vi "Gif.Main.vi"(5 "String":string, 9 "bgcolor":u32(colorbox)=16777226, 11 "error in (no error)":errorcluster, 12 "image index":i32) -> (6 "time":u32[](array[numeric]), 8 "images out":picture[](array[picture]), 13 "image data":T1, 14 "image size":cluster{"Width":u32, "Height":u32}, 15 "error out":errorcluster)   [LabVIEW 2011]
doc: "This VI reads all images from a gif file.\nCurrently it can only read from version 89a.\nInterlaced images are not taken into account.\n\nThe outputs are an array of all delay times, an array of all images, the image size and an error cluster.\n\nVersion 01.01\nMike Schröder"
uses:
  <vilib>/picture/picture.llb/imagedata.ctl
panel:
  out "color table":u32[](array[colorbox])
  out "Version":string
  out "Signature":string
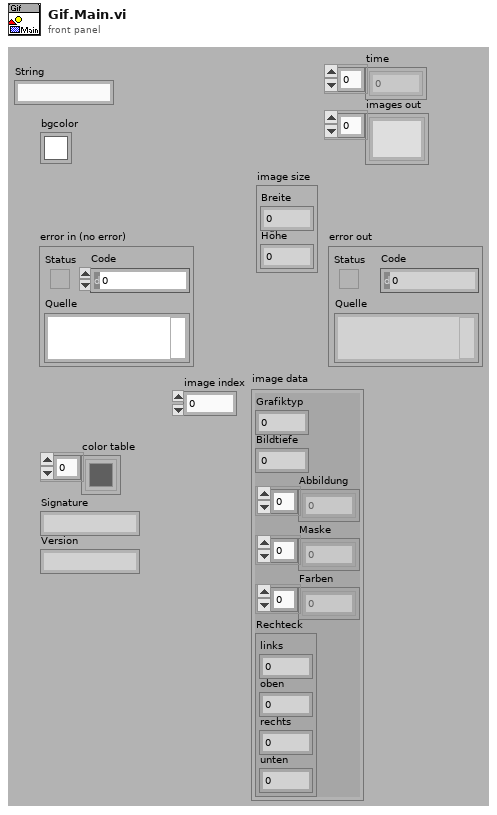
[diagram p1: front panel]
types:
  T1 = typedef "imagedata.ctl" = cluster{"image type":i32, "image depth":i32, "image":u8[], "mask":u8[], "colors":u32[], "Rectangle":cluster{"left":i16, "top":i16, "right":i16, "bottom":i16}}
  T2 = typedef "Gif.LogicalScreenDescriptior.ctl" = cluster{"Logical Screen Width":u16, "Logical Screen Height":u16, "Global Color Table Flag":u8, "Color Resolution":u8, "Sort Flag":u8, "Size of Global Color Table":u8, "Background Color Index":u8, "Pixel Aspect Ratio":u8}
  T3 = typedef "Gif.GraphicControlExtension.ctl" = cluster{"Reserved":u8, "Disposal Method":u8, "User Input Flag":u8, "Transparent Color Flag":u8, "Delay Time":u16, "Transparent Color Index":u8}
  T4 = typedef "Gif.ImageDescriptor.ctl" = cluster{"Image Left Position":u16, "Image Top Position":u16, "Image Width":u16, "Image Height":u16, "Local Color Table Flag":u8, "Interlace Flag":u8, "Sort Flag":u8, "Reserved":u8, "Size Of Local Color Table":u8}
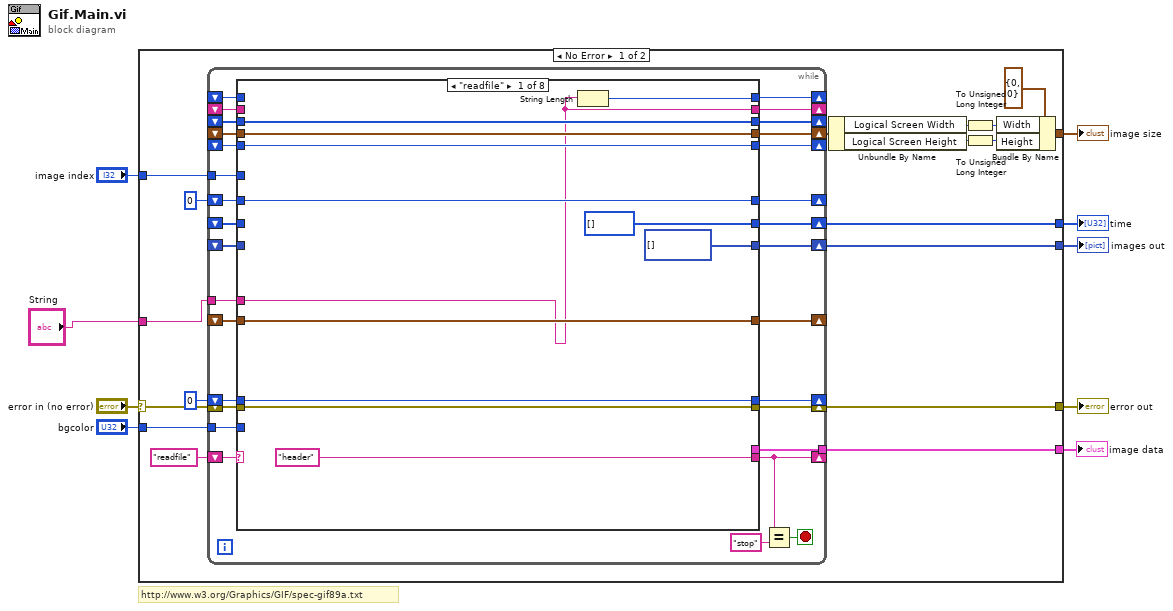
[diagram p0: block diagram]
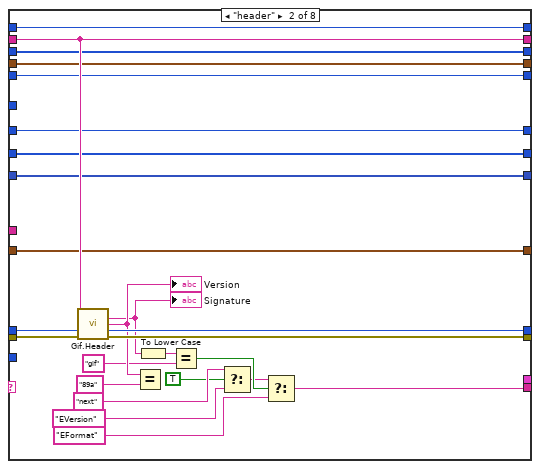
[diagram p2: hidden frame]
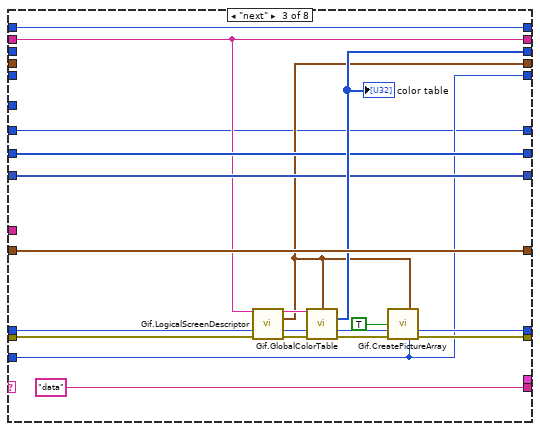
[diagram p3: hidden frame]
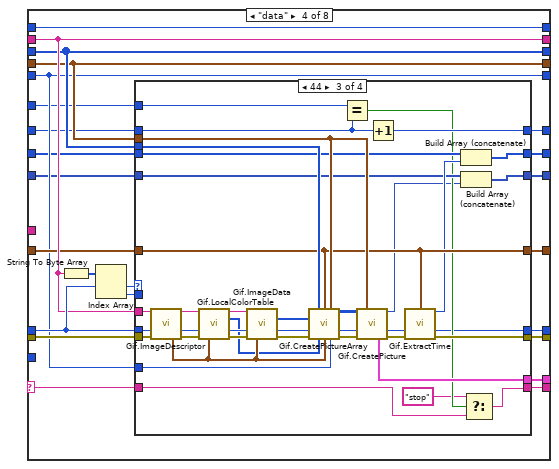
[diagram p4: hidden frame]
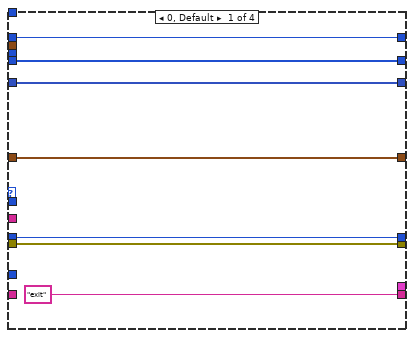
[diagram p5: hidden frame]
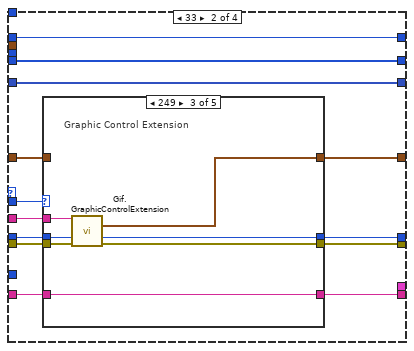
[diagram p6: hidden frame]
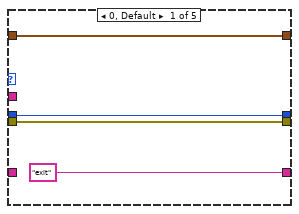
[diagram p7: hidden frame]
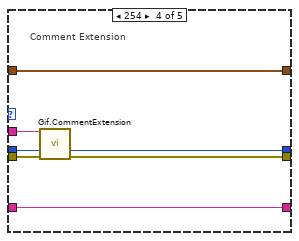
[diagram p9: hidden frame]
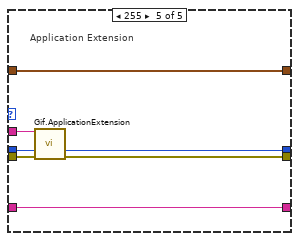
[diagram p10: hidden frame]
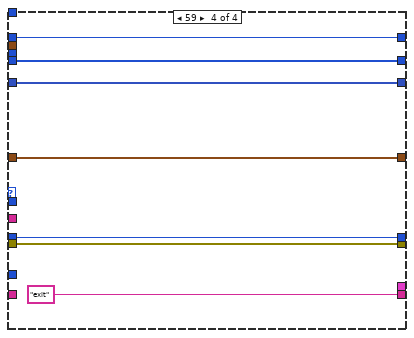
[diagram p11: hidden frame]
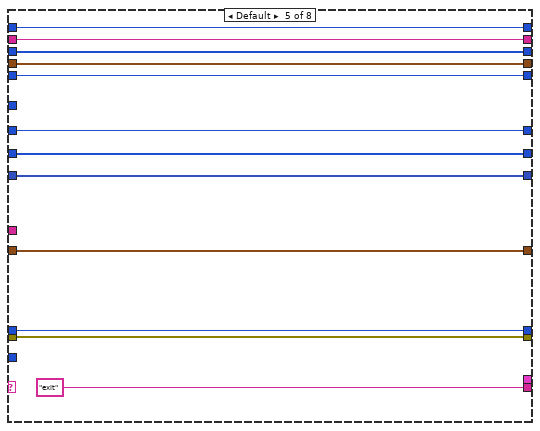
[diagram p12: hidden frame]
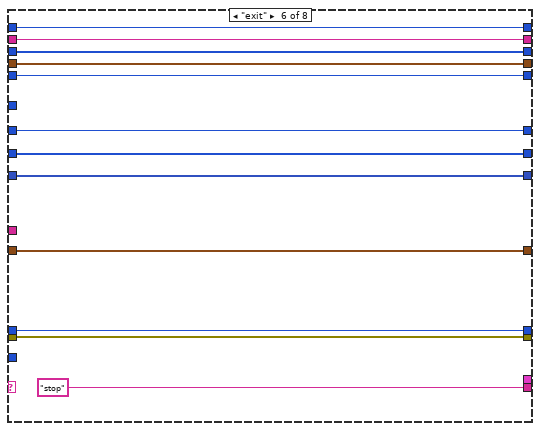
[diagram p13: hidden frame]
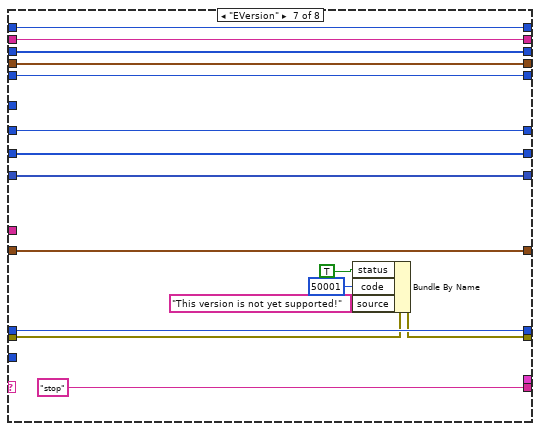
[diagram p14: hidden frame]
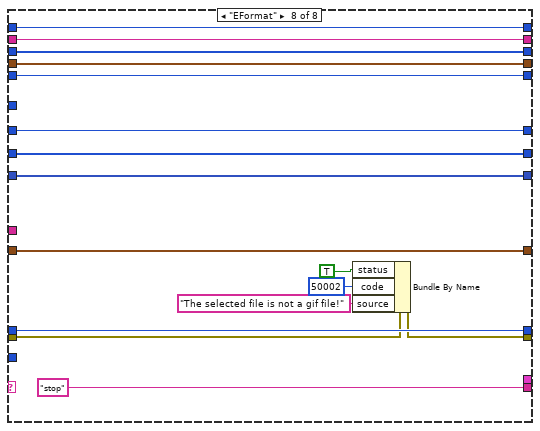
[diagram p15: hidden frame]
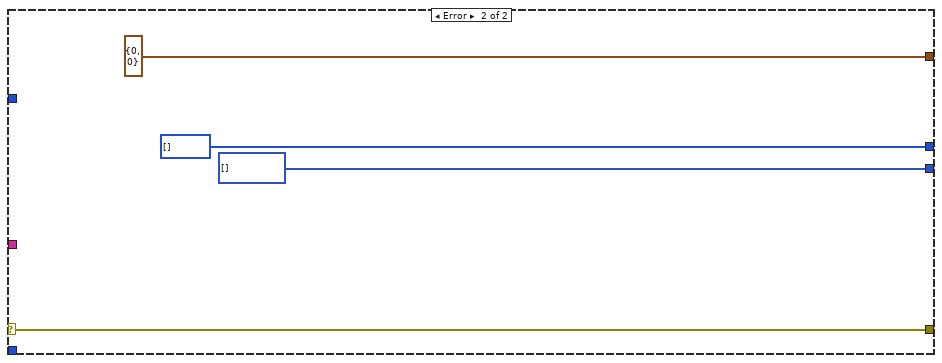
[diagram p16: hidden frame]
diagram:
  # "http://www.w3.org/Graphics/GIF/spec-gif89a.txt"
  n1 = case shown="No Error" "error in (no error)" {
    selector: "error in (no error)" -> [w14 w293]
    tunnel: [w25 u32[] []] -> w9
    tunnel: [w24 picture[] []] -> w2
    tunnel: "bgcolor" -> [w22 _]
    tunnel: [w21 w293] -> w7
    tunnel: [w15 cluster{"Width":u32, "Height":u32} {"Width"=0, "Height"=0} ("Größe des Darstellungsbereichs")] -> w6
    tunnel: "image index" -> [w12 _]
    tunnel: [w11 _] -> w3
    tunnel: "String" -> [w10 _]
    frame No Error {
      n2 = while {
        shift-right: [w48] -> _
        shift-left: "readfile" -> [w57]
        shift-right: [w56] -> _
        shift-left: _ -> [w54]
        shift-right: [w55] -> _
        shift-left: _ -> [w53]
        shift-right: [w51] -> w21
        shift-left: w14 -> [w52]
        shift-right: [w49] -> _
        shift-left: 0 ("offset (0)") -> [w50]
        shift-right: [w45] -> _
        shift-left: _ -> [w44]
        shift-right: [w43] -> _
        shift-left: _ -> [w42]
        shift-right: [w41] -> w23
        shift-left: _ -> [w40]
        shift-right: [w39] -> _
        shift-left: _ -> [w38]
        shift-right: [w36] -> w25
        shift-left: _ -> [w37]
        shift-right: [w34] -> w24
        shift-left: _ -> [w35]
        tunnel: w22 -> [w33]
        shift-right: [w30] -> _
        shift-left: 0 ("offset (0)") -> [w31]
        tunnel: w12 -> [w29]
        tunnel: [w32] -> w11
        tunnel: w10 -> [w28]
        stop <- w46 stop-if-true
        n3 = case shown="\"readfile\"" w57 {
          selector: w57 -> [_ _ _ w129 _ _ _ _]
          tunnel: [w69 w94 w114 w138 w245 w257 w273 w289] -> w56
          tunnel: [w59 w92 w98 w128 w244 w256 w272 w288] -> w55
          tunnel: w54 -> [_ w94 w114 w138 w245 w257 w273 w289]
          tunnel: w53 -> [_ w92 w98 w128 w244 w256 w272 w288]
          tunnel: ["header" w73 "data" w130 "exit" "stop" "stop" "stop"] -> w48
          tunnel: w52 -> [w58 w93 w97 w133 w242 w254 w263 w279]
          tunnel: [w58 w87 w101 w132 w242 w254 w262 w278] -> w51
          tunnel: w50 -> [w67 w91 w96 w134 w241 w253 w270 w286]
          tunnel: [w67 w86 w103 w131 w241 w253 w270 w286] -> w49
          tunnel: [w66 w85 w108 w127 w240 w252 w269 w285] -> w45
          tunnel: w44 -> [w66 w85 _ w127 w240 w252 w269 w285]
          tunnel: [w65 w90 w112 w126 w239 w251 w268 w284] -> w43
          tunnel: w42 -> [w65 w90 w112 w125 w239 w251 w268 w284]
          tunnel: [w64 w84 w100 w124 w238 w250 w267 w283] -> w41
          tunnel: w40 -> [w64 w84 _ w124 w238 w250 w267 w283]
          tunnel: [w63 w83 w99 w123 w237 w249 w266 w282] -> w39
          tunnel: w38 -> [w63 w83 _ w123 w237 w249 w266 w282]
          tunnel: w37 -> [_ w89 w107 w122 w236 w248 w265 w281]
          tunnel: [u32[] [] w89 w107 w121 w236 w248 w265 w281] -> w36
          tunnel: w35 -> [_ w88 w106 w120 w235 w247 w264 w280]
          tunnel: [picture[] [] w88 w106 w119 w235 w247 w264 w280] -> w34
          tunnel: w33 -> [_ _ w99 _ _ _ _ _]
          tunnel: [_ _ _ w118 _ _ _ _] -> w32
          tunnel: w31 -> [w61 w70 w95 w117 w234 w246 w258 w274]
          tunnel: [w61 w70 w95 w116 w234 w246 w258 w274] -> w30
          tunnel: w29 -> [_ _ _ w115 _ _ _ _]
          tunnel: w28 -> [w59 _ _ _ _ _ _ _]
          frame "readfile" {
            n4 = String Length(string=w59) -> (length=w69:i32)
          }
          frame "header" {
            n5 = call "Gif.Header.vi"("data"=w92, "offset"=w91, "error in (no error)"=w93) -> ("Signature"=w78:string, "Version"=w82:string, "offset out"=w86:i32, "error out"=w87:errorcluster)  [unwired: 1 in, 8 out]
            "Signature" <- w78
            "Version" <- w82
            n6 = Equal?(x=w82, y="89a") -> ()  [unwired: 1 out]
            n7 = To Lower Case(string=w78) -> (all lower case string=w77:string)
            n8 = Equal?(x=w77, y="gif") -> (x = y?=w75:bool)
            n9 = Select(t="next", s=TRUE, f="EVersion") -> (s? t:f=w74:string)
            n10 = Select(t=w74, s=w75, f="EFormat") -> (s? t:f=w73:string)
          }
          frame "next" {
            n11 = call "Gif.LogicalScreenDescriptor.vi"("data"=w98, "offset"=w96, "error in (no error)"=w97) -> ("data out"=w109:string, "Logical Screen Descriptor"=w100:T2, "offset out"=w110:i32, "error out"=w111:errorcluster)  [unwired: 9 out]
            n12 = call "Gif.GlobalColorTable.vi"("data"=w109, "Logical Screen Descriptor"=w100, "offset"=w110, "error in (no error)"=w111) -> ("global color table"=w108:u32[], "offset out"=w104:i32, "error out"=w102:errorcluster)  [unwired: 1 in, 8 out]
            "color table" <- w108
            n13 = call "Gif.CreatePictureArray.vi"("Logical Screen Description"=w100, "init"=TRUE, "offset"=w104, "error in (no error)"=w102, "bgcolor"=w99) -> ("offset out"=w103:i32, "error out"=w101:errorcluster)  [unwired: 5 in, 4 out]
          }
          frame "data" {
            n14 = String To Byte Array(string=w128) -> (unsigned byte array=w137:u8[])
            n15 = Index Array(array=w137, index #1=w134) -> (element #1=w136:u8, element #2=w135:u8)  [unwired: 1 in]
            n16 = case shown="44" w136 {
              tunnel: w135 -> [_ w158 _ _]
              tunnel: w134 -> [w144 w154 w225 w232]
              tunnel: w133 -> [w145 w153 w226 w231]
              tunnel: [w145 w152 w200 w231] -> w132
              tunnel: [w144 w155 w190 w232] -> w131
              tunnel: ["exit" w157 w192 "exit"] -> w130
              tunnel: w129 -> [_ w156 w194 _]
              tunnel: w128 -> [_ w151 w224 _]
              tunnel: w127 -> [_ _ w210 _]
              tunnel: [w142 w150 w208 w230] -> w126
              tunnel: w125 -> [w142 w149 w208 w230]
              tunnel: w124 -> [_ _ w209 _]
              tunnel: w123 -> [_ _ w207 _]
              tunnel: w122 -> [w141 w148 w206 w229]
              tunnel: [w141 w148 w204 w229] -> w121
              tunnel: w120 -> [w140 w147 w203 w228]
              tunnel: [w140 w147 w202 w228] -> w119
              tunnel: [_ _ w198 _] -> w118
              tunnel: w117 -> [w139 w146 w188 w227]
              tunnel: [w139 w146 w196 w227] -> w116
              tunnel: w115 -> [_ _ w197 _]
              frame 0, Default {
              }
              frame 33 {
                n17 = case shown="249" w158 {
                  tunnel: ["exit" w166 w173 w180 w187] -> w157
                  tunnel: w156 -> [_ w166 w173 w180 w187]
                  tunnel: [w161 w165 w169 w177 w185] -> w155
                  tunnel: w154 -> [w161 w165 w171 w178 w186]
                  tunnel: w153 -> [w160 w164 w172 w179 w184]
                  tunnel: [w160 w164 w170 w176 w183] -> w152
                  tunnel: w151 -> [_ _ w168 w175 w182]
                  tunnel: [w159 w163 w167 w174 w181] -> w150
                  tunnel: w149 -> [w159 w163 _ w174 w181]
                  frame 0, Default {
                  }
                  frame 1 {
                  }
                  frame 249 {
                    # "Graphic Control Extension"
                    n18 = call "Gif.GraphicControlExtension.vi"("data"=w168, "offset"=w171, "error in (no error)"=w172) -> ("GraphicControlExtension"=w167:T3, "offset out"=w169:i32, "error out"=w170:errorcluster)  [unwired: 10 out]
                  }
                  frame 254 {
                    # "Comment Extension"
                    n19 = call "Gif.CommentExtension.vi"("data"=w175, "offset"=w178, "error in (no error)"=w179) -> ("offset out"=w177:i32, "error out"=w176:errorcluster)  [unwired: 11 out]
                  }
                  frame 255 {
                    # "Application Extension"
                    n20 = call "Gif.ApplicationExtension.vi"("data"=w182, "offset"=w186, "error in (no error)"=w184) -> ("offset out"=w185:i32, "error out"=w183:errorcluster)  [unwired: 11 out]
                  }
                }
              }
              frame 44 {
                n21 = call "Gif.ImageDescriptor.vi"("data"=w224, "offset"=w225, "error in (no error)"=w226) -> ("data out"=w221:string, "offset out"=w222:i32, "ImageDescriptor"=w212:T4, "error out"=w223:errorcluster)  [unwired: 9 out]
                n22 = call "Gif.LocalColorTable.vi"("data"=w221, "offset"=w222, "error in (no error)"=w223, "ImageDescriptor"=w212) -> ("data out"=w218:string, "local color table"=w211:u32[], "offset out"=w219:i32, "error out"=w220:errorcluster)  [unwired: 5 in, 3 out]
                n23 = call "Gif.ImageData.vi"("data"=w218, "offset"=w219, "error in (no error)"=w220, "ImageDescriptor"=w212) -> ("Index Array"=w216:i32[], "offset out"=w191:i32, "error out"=w217:errorcluster)  [unwired: 1 in, 8 out]
                n24 = call "Gif.CreatePictureArray.vi"("gloal color table"=w210, "GraphicControlExtension"=w208, "Logical Screen Description"=w209, "Index Array"=w216, "offset"=w191, "error in (no error)"=w217, "local color table"=w211, "ImageDescriptor"=w212, "bgcolor"=w207) -> ("image out"=w213:u32[][], "offset out"=w214:i32, "error out"=w215:errorcluster)  [unwired: 1 in, 3 out]
                n25 = Equal?(x=w197, y=w188) -> (x = y?=w195:bool)
                n26 = call "Gif.CreatePicture.vi"("image in"=w213, "Logical Screen Description"=w209, "offset"=w214, "error in (no error)"=w215) -> ("image out"=w189:picture, "offset out"=w199:i32, "graphic data"=w198:T1, "error out"=w201:errorcluster)  [unwired: 8 out]
                n27 = Increment(x=w188) -> (x+1=w196:i32)
                n28 = call "Gif.ExtractTime.vi"("GraphicControlExtension"=w208, "offset"=w199, "error in (no error)"=w201) -> ("time"=w205:u32, "offset out"=w190:i32, "error out"=w200:errorcluster)  [unwired: 10 out]
                n29 = Build Array (concatenate)(w206, w205) -> (w204:u32[])
                n30 = Build Array (concatenate)(w203, w189) -> (w202:picture[])
                n31 = Select(t="stop", s=w195, f=w194) -> (s? t:f=w192:string)
              }
              frame 59 {
              }
            }
          }
          frame Default {
          }
          frame "exit" {
          }
          frame "EVersion" {
            n32 = Bundle By Name(cluster=w263, "status"=TRUE, "code"=50001, "source"="This version is not yet supported!") -> (w262:errorcluster)
          }
          frame "EFormat" {
            n33 = Bundle By Name(cluster=w279, "status"=TRUE, "code"=50002, "source"="The selected file is not a gif file!") -> (w278:errorcluster)
          }
        }
        n34 = Equal?(x=w48, y="stop") -> (x = y?=w46:bool)
      }
      n35 = Unbundle By Name(w23) -> ("Logical Screen Width"=w18:u16, "Logical Screen Height"=w17:u16)
      n36 = To Unsigned Long Integer(number=w18) -> (unsigned 32bit integer=w19:u32)
      n37 = To Unsigned Long Integer(number=w17) -> (unsigned 32bit integer=w20:u32)
      n38 = Bundle By Name(cluster=cluster{"Width":u32, "Height":u32} {"Width"=0, "Height"=0} ("Größe des Darstellungsbereichs"), "Width"=w19, "Height"=w20) -> (w15:cluster{"Width":u32, "Height":u32})
    }
    frame Error {
    }
  }
  "time" <- w9
  "error out" <- w7
  "image size" <- w6
  "image data" <- w3
  "images out" <- w2
